vi "Fetch Measurement (Time Voltage Interval).vi"(0 "VISA resource name":refnum<visa-resource-name>, 1 "Slope (0: Positive)":i32(ring) items=["Positive", "Negative"], 2 "Occurrence (3)":i32=3 format="%.0g", 5 "Channel (1: Channel 1)":i32(ring)=1 items=["Channel 1"=1, "Channel 2"=2, "Channel 3"=3, "Channel 4"=4, "Function 1"=5, "Function 2"=6, "Function 3"=7, "Function 4"=8, "Memory 1"=9, "Memory 2"=10, "Memory 3"=11, "Memory 4"=12], 7 "Voltage Level (-0.25)":dbl=-0.25, 11 "error in (no error)":errorcluster) -> (4 "VISA resource name out":refnum<visa-resource-name>, 6 "Time Interval (s)":dbl, 15 "error out":errorcluster)   [LabVIEW 2009, in "Agilent 8000 Series.lvlib"]
doc: "Obtains a waveform measurement (Time Voltage Interval) and returns the measurement value. The waveform on which the oscilloscope calculates the waveform measurement is from an acquisition that you previously initiated. \n\nUse the Initiate Acquisition.vi to start an acquisition on the channels that you enable with the Configure Channel.vi. The oscilloscope acquires waveforms for the enabled channels concurrently. You use the Wait For Operation Complete.vi to wait for operation complete. You call this VI separately for each waveform measurement you want to obtain on a specific channel.\n\nYou can call the Read Measurement.vi instead of the Initiate Acquisition.vi. The Read Measurement.vi starts an acquisition on all enabled channels. It then waits for the acquisition to complete, obtains a waveform measurement on the channel you specify, and returns the measurement value. You call this VI separately for any other waveform measurement that you want to obtain on a specific channel.\n\nNotes:\n\n(1) You must configure the appropriate reference levels before you call this VI to take measurement.\n\n(2) You configure the low, mid, and high references either by calling the Configure Reference Levels.vi.\n\n(3) This VI does not check the instrument status. Typically, you call this VI only in a sequence of calls to other low-level driver VIs. The sequence performs one operation. You use the low-level VIs to optimize one or more aspects of interaction with the instrument. If you want to check the instrument status, call the Error-Query.vi at the conclusion of the sequence."
uses:
  Agilent 8000 Series.lvlib
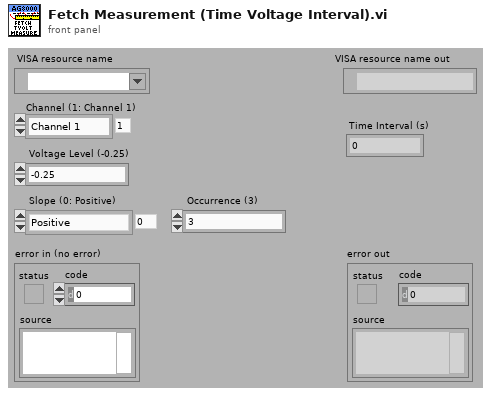
[diagram p1: front panel]
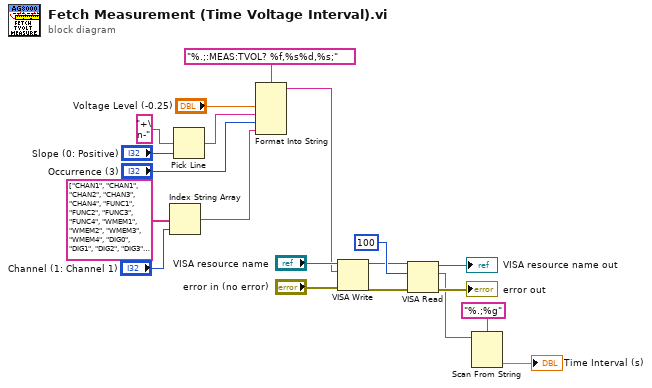
[diagram p0: block diagram]
diagram:
  n1 = Index String Array(1:"Channel (1: Channel 1)", 2:string[] ["CHAN1", "CHAN1", "CHAN2", "CHAN3", "CHAN4", "FUNC1", "FUNC2", "FUNC3", "FUNC4", "WMEM1", "WMEM2", "WMEM3", "WMEM4", "DIG0", "DIG1", "DIG2", "DIG3", "DIG4", "DIG5", "DIG6", "DIG7", "DIG8", "DIG9", "DIG10", "DIG11", "DIG12", "DIG13", "DIG14", "DIG15", "AUX", "LINE"]) -> (0:w12:string)  [unwired: 1 in]
  n2 = Pick Line(multi-line string="+\n-", line index="Slope (0: Positive)") -> (output string=w14:string)  [unwired: 1 in]
  n3 = Format Into String(format string="%.;:MEAS:TVOL? %f,%s%d,%s;", "Voltage Level (-0.25)", w14, "Occurrence (3)", w12) -> (resulting string=w4:string)  [unwired: 2 in, 1 out]
  n4 = VISA Write(VISA resource name="VISA resource name", write buffer=w4, error in (no error)="error in (no error)") -> (VISA resource name out=w8:refnum<visa-resource-name>, error out=w9:errorcluster)  [unwired: 1 out]
  n5 = VISA Read(VISA resource name=w8, byte count=u32 100, error in (no error)=w9) -> (VISA resource name out=→"VISA resource name out":refnum<visa-resource-name>, read buffer=w1:string, error out=→"error out":errorcluster)  [unwired: 1 out]
  n6 = Scan From String(format string="%.;%g", input string=w1) -> (output 1=→"Time Interval (s)":dbl)  [unwired: 3 in, 3 out]
